vi "Update Input Graph.vi"() -> ()   [LabVIEW 2021, in "User Interface.lvlib"]
uses:
  User Interface.lvlib
panel:
  out "Legend:Number of Rows":u32
  out "Waveform Chart":T1(graph)
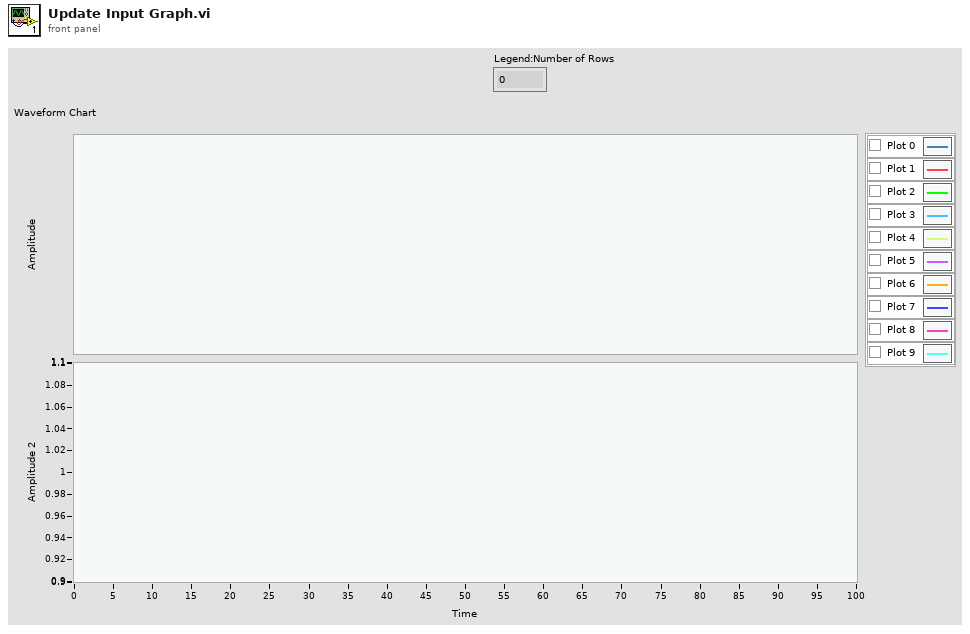
[diagram p1: front panel]
types:
  T1 = cluster{"Legend:Number of Rows":u32, "Legend:Number of Rows":u32}
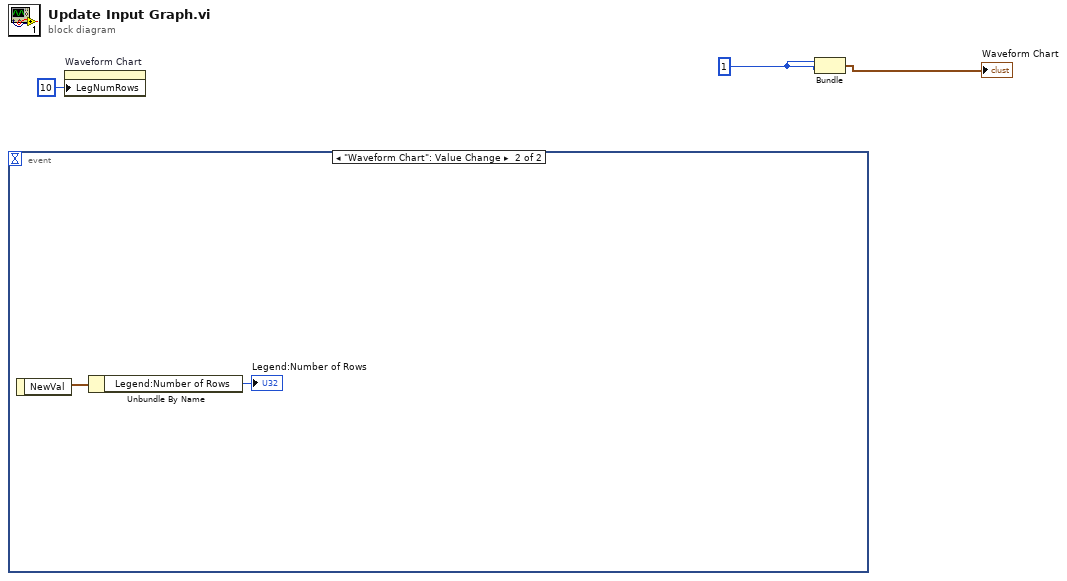
[diagram p0: block diagram]
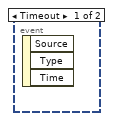
[diagram p2: hidden frame]
diagram:
  w2 = u32 1 ("Legend:Number of Rows")
  n1 = event shown="[1] \"Waveform Chart\": Value Change" {
    selector: _ -> [_ _]
    dyn-events: _ -> [_ _]
    timeout: _ -> [_ _]
    event Timeout {
      n2 = event-data() -> ()  [unwired: 1 in, 3 out]
    }
    event "Waveform Chart": Value Change {
      n3 = event-data() -> ("NewVal"=w5:T1)  [unwired: 1 in]
      n4 = Unbundle By Name(w5) -> ("Legend:Number of Rows"=→"Legend:Number of Rows":u32)
    }
  }
  n5 = property on="Waveform Chart" class="WFChart (strict)"("LegNumRows"=u32 10 ("Legend:Number of Rows")) -> ()  [unwired: 2 in, 2 out]
  n6 = Bundle("Legend:Number of Rows"=w2, "Legend:Number of Rows"=w2) -> (→"Waveform Chart":T1)  [unwired: 1 in]
